vi "Get Tach RPM (FPGA).vi"(8 "Pulses/Revolution":sgl=2.0, 9 "Threshold Settings":T2={"threshold"=0.0, "hysteresis"=0.0, "slope (rising)"=enum."rising"}, 10 "Max Tach Period (uSec)":u32=1000000, 11 "Analog Tach Signal":fxp<+/-,24,4>) -> (1 "Tach State":T1, 2 "Tach RPM":sgl)   [LabVIEW 2014, in "Tachometer (SGL).lvlib"]
uses:
  Tachometer (SGL).lvlib
  Threshold Settings.ctl
  Tach State.ctl
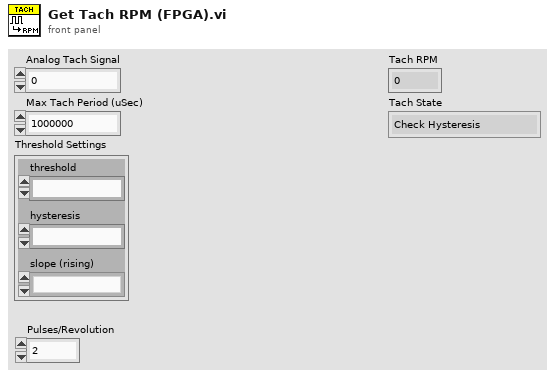
[diagram p1: front panel]
types:
  T1 = typedef "Tachometer (SGL).lvlib/Tach State.ctl" = enum16{"Check Hysteresis", "Check Threshold"}
  T2 = typedef "Tachometer (SGL).lvlib/Threshold Settings.ctl" = cluster{"threshold":fxp<+/-,24,4>, "hysteresis":fxp<+/-,24,4>, "slope (rising)":enum16{"falling", "rising"}}
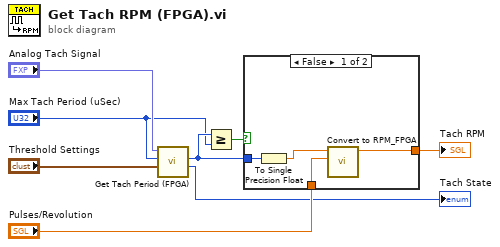
[diagram p0: block diagram]
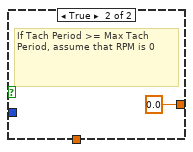
[diagram p2: hidden frame]
diagram:
  n1 = call "Get Tach Period (FPGA).vi"("Threshold Settings"="Threshold Settings", "Max Tach Period (uSec)"="Max Tach Period (uSec)", "Analog Tach Signal"="Analog Tach Signal") -> ("Tach State"=→"Tach State":T1, "Tach Period (uSec/pulse)"=w3:u32)  [unwired: 7 in]
  n2 = Greater Or Equal?(x=w3, y="Max Tach Period (uSec)") -> (x >= y?=w1:bool)
  n3 = case shown="False" w1 {
    tunnel: "Pulses/Revolution" -> [w11 _]
    tunnel: [w10 sgl 0.0 ("Tach RPM")] -> w5
    tunnel: w3 -> [w9 _]
    frame False {
      n4 = To Single Precision Float(number=w9) -> (single precision float=w12:sgl)
      n5 = call "Convert to RPM_FPGA.vi"("pulses/revolution"=w11, "Tach Period (uSec/pulse)"=w12) -> ("Tach RPM"=w10:sgl)  [unwired: 9 in]
    }
    frame True {
      # "If Tach Period >= Max Tach Period, assume that RPM is 0"
    }
  }
  "Tach RPM" <- w5
